vi "ConfigRefClkSource.vi"(8 "error in (no error)":errorcluster, 11 "ClassIn":refnum<class "Keysight335XX.lvclass">) -> (0 "error out":errorcluster, 3 "ClassOut":refnum<class "Keysight335XX.lvclass">)   [LabVIEW 2014, in "FGenPlugins.lvlib" / "Keysight335XX.lvclass"]
uses:
  Keysight335XX.lvclass
  <instrlib>/Agilent 3352X Series/Agilent 3352X Series.lvlib
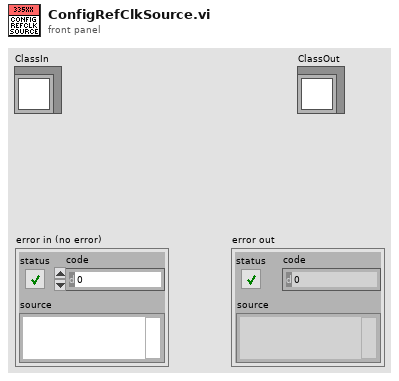
[diagram p1: front panel]
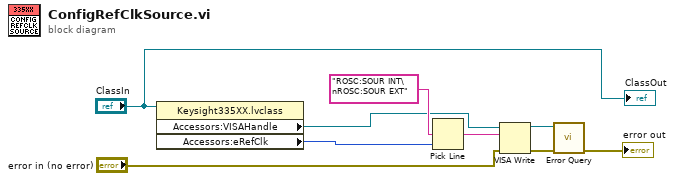
[diagram p0: block diagram]
diagram:
  n1 = property class="Keysight335XX.lvclass"(reference="ClassIn") -> ("Accessors:VISAHandle"=w4:refnum<visa-resource-name>, "Accessors:eRefClk"=w8:u16)  [unwired: 1 in, 2 out]
  n2 = Pick Line(multi-line string="ROSC:SOUR INT\nROSC:SOUR EXT", line index=w8) -> (output string=w5:string)  [unwired: 1 out]
  n3 = VISA Write(VISA resource name=w4, write buffer=w5, error in (no error)="error in (no error)") -> (VISA resource name out=w7:refnum<visa-resource-name>, error out=w6:errorcluster)  [unwired: 1 out]
  n4 = call <instrlib>:"Error Query.vi"("error in (no error)"=w6, "VISA resource name"=w7) -> ("error out"=→"error out":errorcluster)  [unwired: 9 out]
  "ClassOut" <- "ClassIn"
